vi "Vision Processing.vi"(4 "error in (no error)":errorcluster) -> ()   [LabVIEW 2016]
doc: "This VI runs in parallel to other tasks. It gets images from the camera, processes them for color or shape and use that information to affect robot behavior."
uses:
  <vilib>/Rock Robotics/WPI/Camera/WPI_CameraImageSize.ctl
  <vilib>/Rock Robotics/WPI/Camera/WPI_CameraWhite Balance Values.ctl
  <vilib>/Rock Robotics/WPI/Camera/WPI_CameraExposure Values.ctl
  <vilib>/Rock Robotics/WPI/Camera/WPI_CameraFrameRate.ctl
  Robot Global Data.vi
  distance to target.vi
  Global distance.vi
panel:
  out "YP":dbl
  out "d":dbl
  out "Image Size 2":T1
  out "Image":T2(plugin-control)
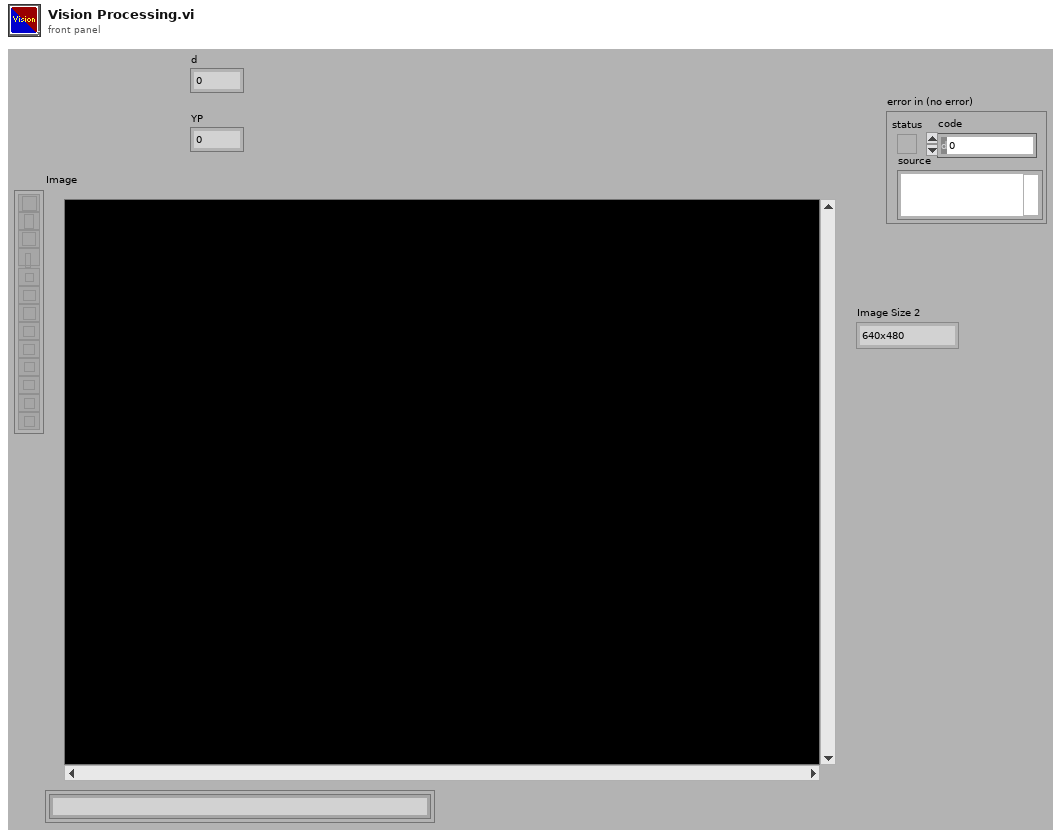
[diagram p1: front panel]
types:
  T1 = typedef "WPI_CameraImageSize.ctl" = enum16{"640x480", "320x240", "160x120", "Custom"}
  T2 = typedef "IMAQ Image.ctl" = refnum<image>
  T3 = typedef "WPI_CameraFrameRate.ctl" = u32
  T4 = typedef "WPI_CameraExposure Values.ctl" = enum16{"Auto", "Flicker-free 50 Hz", "Flicker-free 60 Hz", "Hold current", "Custom"}
  T5 = typedef "WPI_CameraWhite Balance Values.ctl" = enum16{"Auto", "Fixed indoor", "Fixed outdoor 1", "Fixed outdoor 2", "Fixed fluorescent 1", "Fixed fluorescent 2", "Hold current", "Custom"}
  T6 = typedef "Image Type" = u32
  T7 = typedef "WPI_CameraDevRef.ctl" = cluster{"Camera Address":string, "CameraStatus":errorcluster}
  T8 = cluster{"Particle Measurements (Pixels) (find y pixel)[0]":dbl, "Particle Measurements (Pixels) (find y pixel)[1]":dbl, "Particle Measurements (Pixels) (find y pixel)[2]":dbl, "Particle Measurements (Pixels) (find y pixel)[3]":dbl, "Particle Measurements (Pixels) (find y pixel)[4]":dbl, "Particle Measurements (Pixels) (find y pixel)[5]":dbl, "Particle Measurements (Pixels) (find y pixel)[6]":dbl, "Particle Measurements (Pixels) (find y pixel)[7]":dbl, "Particle Measurements (Pixels) (find y pixel)[8]":dbl}
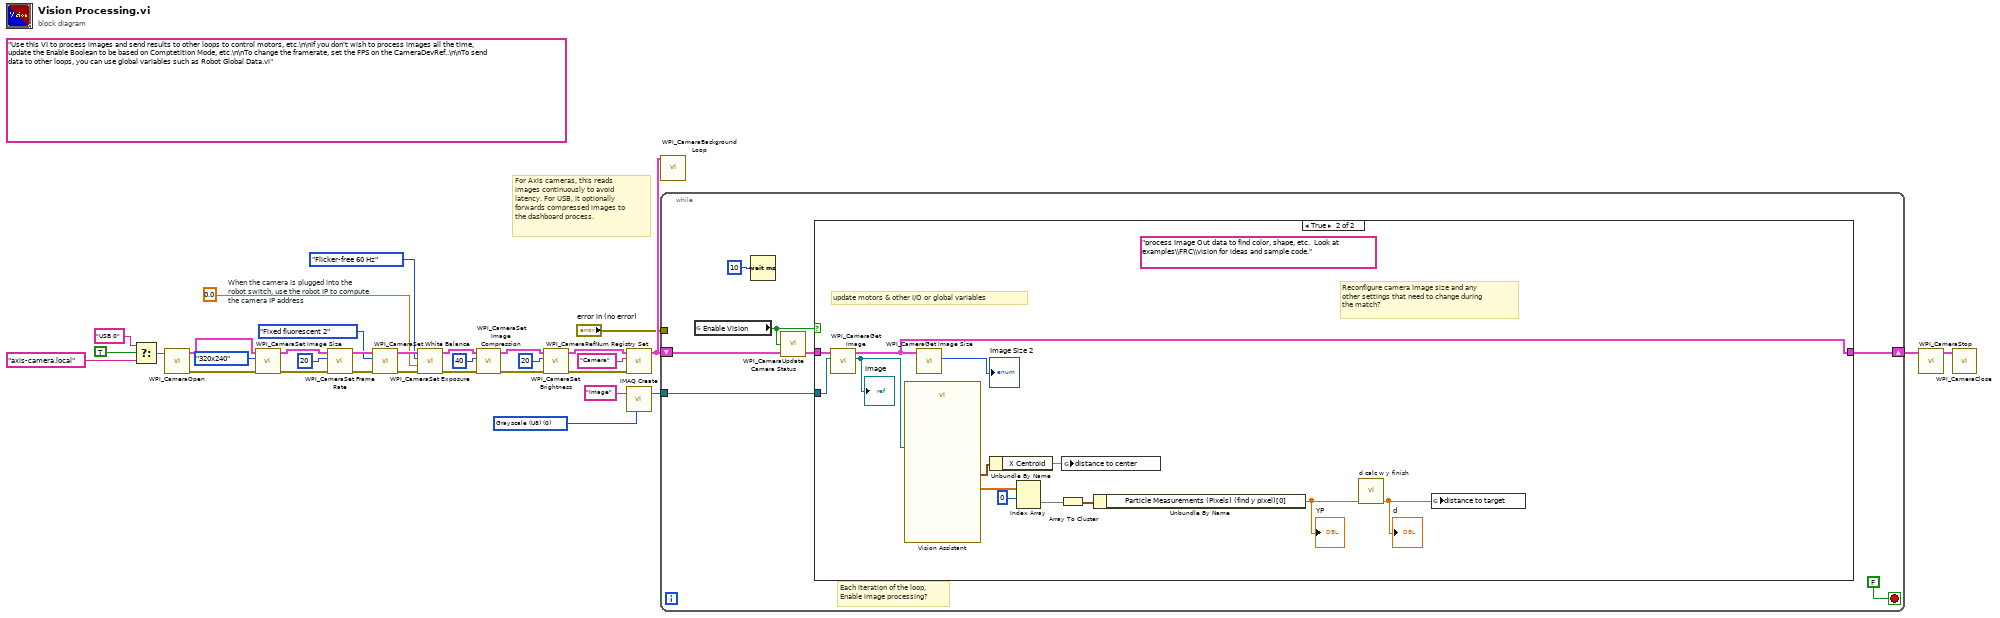
[diagram p0: block diagram]
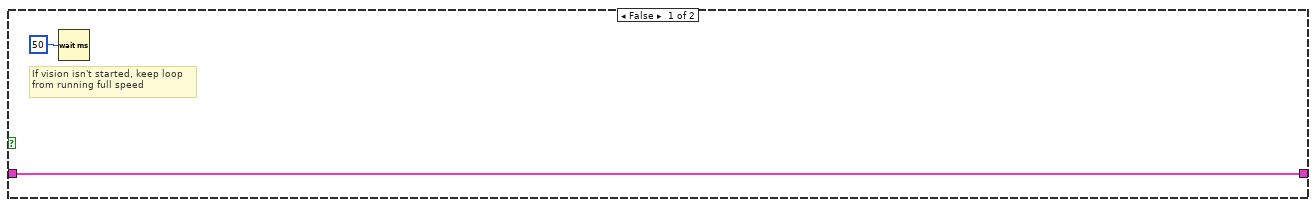
[diagram p2: hidden frame]
diagram:
  (unwired) "Use this VI to process images and send results to other loops to control motors, etc.\n\nIf you don't wish to process images all the time, update the Enable Boolean to be based on Comptetition Mode, etc.\n\nTo change the framerate, set the FPS on the CameraDevRef..\n\nTo send data to other loops, you can use global variables such as Robot Global Data.vi"
  w33 = T6 0 items=["Grayscale (U8)", "Grayscale (I16)", "Grayscale (SGL)", "Complex (CSG)", "RGB (U32)", "HSL (U32)", "RGB (U64)"] ("Image Type")
  # "When the camera is plugged into the\nrobot switch, use the robot IP to compute\nthe camera IP address"
  # "For Axis cameras, this reads\nimages continuously to avoid\nlatency. For USB, it optionally\nforwards compressed images to\nthe dashboard process."
  n1 = Select(t="USB 0" ("format string"), s=TRUE ("dot notation? (F)"), f="axis-camera.local" ("format string")) -> (s? t:f=w8:string)
  n2 = call <vilib>:"WPI_CameraOpen.vi"("Camera Address"=w8) -> ("error out"=w21:errorcluster, "CameraDevRef"=w22:T7)  [unwired: 1 in, 8 out]
  n3 = call <vilib>:"WPI_CameraSet Image Size.vi"("error in (no error)"=w21, "Image Size"=WPI_CameraImageSize."320x240", "CameraDevRef"=w22) -> ("error out"=w20:errorcluster, "CameraDevRef Out"=w23:T7)  [unwired: 1 in, 6 out]
  n4 = call <vilib>:"WPI_CameraSet Frame Rate.vi"("error in (no error)"=w20, "Frame Rate (fps)"=T3 20, "CameraDevRef"=w23) -> ("error out"=w19:errorcluster, "CameraDevRef Out"=w25:T7)  [unwired: 7 out]
  n5 = call <vilib>:"WPI_CameraSet White Balance.vi"("error in (no error)"=w19, "White Balance"=WPI_CameraWhite_Balance_Values."Fixed fluorescent 2", "CameraDevRef"=w25) -> ("error out"=w18:errorcluster, "CameraDevRef Out"=w24:T7)  [unwired: 1 in, 6 out]
  n6 = call <vilib>:"WPI_CameraSet Exposure.vi"("error in (no error)"=w18, "Exposure (%)"=0.0, "Exposure"=WPI_CameraExposure_Values."Flicker-free 60 Hz", "CameraDevRef"=w24) -> ("error out"=w17:errorcluster, "CameraDevRef Out"=w27:T7)  [unwired: 6 out]
  n7 = call <vilib>:"WPI_CameraSet Image Compression.vi"("error in (no error)"=w17, "Compression"=40, "CameraDevRef"=w27) -> ("error out"=w16:errorcluster, "CameraDevRef Out"=w26:T7)  [unwired: 7 out]
  n8 = call <vilib>:"WPI_CameraSet Brightness.vi"("error in (no error)"=w16, "Brightness"=20, "CameraDevRef"=w26) -> ("error out"=w4:errorcluster, "CameraDevRef Out"=w5:T7)  [unwired: 7 out]
  n9 = call <vilib>:"WPI_CameraRefNum Registry Set.vi"("error in (no error)"=w4, "refnum name"="Camera", "CameraDevRef"=w5) -> ("CameraDevRef"=w12:T7)  [unwired: 1 in, 7 out]
  n10 = call "IMAQ Create"("Image Name"="Image", "Image Type"=w33) -> ("New Image"=w31:T2)  [unwired: 2 in, 2 out]
  n11 = call <vilib>:"WPI_CameraBackground Loop.vi"("CameraDevRef"=w12) -> ()  [unwired: 11 in]
  n12 = while {
    shift-right: [w39] -> w3
    shift-left: w12 -> [w38]
    tunnel: w31 -> [w35]
    tunnel: "error in (no error)" -> [_]
    stop <- FALSE stop-if-true
    # "Each iteration of the loop,\nEnable image processing?"
    n13 = global read "Robot Global Data.vi" "Enable Vision"() -> (w36:bool)
    n14 = Wait (ms)(milliseconds to wait=u32 10) -> ()  [unwired: 1 out]
    n15 = call <vilib>:"WPI_CameraUpdate Camera Status.vi"("CameraDevRef In"=w38, "Enable Vision"=w36) -> ("CameraDevRef Out"=w37:T7)  [unwired: 3 in]
    n16 = case shown="True" w36 {
      tunnel: [w42 w53] -> w39
      tunnel: w37 -> [w42 w55]
      tunnel: w35 -> [_ w54]
      frame False {
        # "If vision isn't started, keep loop\nfrom running full speed"
        n17 = Wait (ms)(milliseconds to wait=u32 50) -> ()  [unwired: 1 out]
      }
      frame True {
        (unwired) "process Image Out data to find color, shape, etc.  Look at examples\\FRC\\vision for ideas and sample code."
        # "update motors & other I/O or global variables"
        # "Reconfigure camera image size and any\nother settings that need to change during\nthe match?"
        n18 = call <vilib>:"WPI_CameraGet Image.vi"("Image"=w54, "CameraDevRef"=w55) -> ("Image Out"=w49:T2, "CameraDevRef Out"=w53:T7)  [unwired: 1 in, 7 out]
        "Image" <- w49
        n19 = call "Vision Assistant"("Image In"=w49) -> ("Centroid (find center)"=w51:cluster{"X Centroid":sgl, "Y Centroid":sgl}, "Particle Measurements (Pixels) (find y pixel)"=w48:dbl[][])  [unwired: 21 in, 4 out]
        n20 = call <vilib>:"WPI_CameraGet Image Size.vi"("CameraDevRef"=w53) -> ("Image Size"=→"Image Size 2":T1)  [unwired: 7 in, 3 out]
        n21 = Unbundle By Name(w51) -> ("X Centroid"=w43:sgl)
        n22 = Index Array(array=w48, index (row)=0) -> (element=w46:dbl[])  [unwired: 1 in]
        n23 = Array To Cluster(array=w46) -> (cluster=w45:T8)
        n24 = global write "Global distance.vi" "distance to center"(w43) -> ()
        n25 = Unbundle By Name(w45) -> ("Particle Measurements (Pixels) (find y pixel)[0]"=w44:dbl)
        "YP" <- w44
        n26 = call "d calc w y finish.vi"("YP"=w44) -> ("d"=w50:dbl)  [unwired: 6 in]
        "d" <- w50
        n27 = global write "distance to target.vi" "distance to target"(w50) -> ()
      }
    }
  }
  n28 = call <vilib>:"WPI_CameraStop.vi"("CameraDevRef"=w3) -> ("CameraDevRef"=w2:T7)  [unwired: 9 in, 1 out]
  n29 = call <vilib>:"WPI_CameraClose.vi"("CameraDevRef"=w2) -> ()  [unwired: 1 in, 10 out]
